vi "image process.vi"(0 "Picture in":refnum<vi>, 1 "reference in":refnum<vi>, 4 "XYGraph Refnum":refnum<vi>, 5 "error in (no error)":errorcluster, 6 "Konverziós faktor":i32 min=0 max=16777215, 7 "picture in":path, 8 "Szürkeárnyalat":i32) -> (10 "new picture 3":picture, 11 "scale maximum":u32, 12 "régi y felbontás":i16, 13 "átméretezett kép":i32[][](array[numeric]), 14 "régi x felbontás":i16, 15 "új y felbontás / sorok száma":i32, 16 "új x felbontás / oszlopok száma":i32, 17 "new picture 2":picture, 19 "error out":errorcluster)   [LabVIEW 2016]
uses:
  <vilib>/Utility/miscctls.llb/LVBoundsTypeDef.ctl
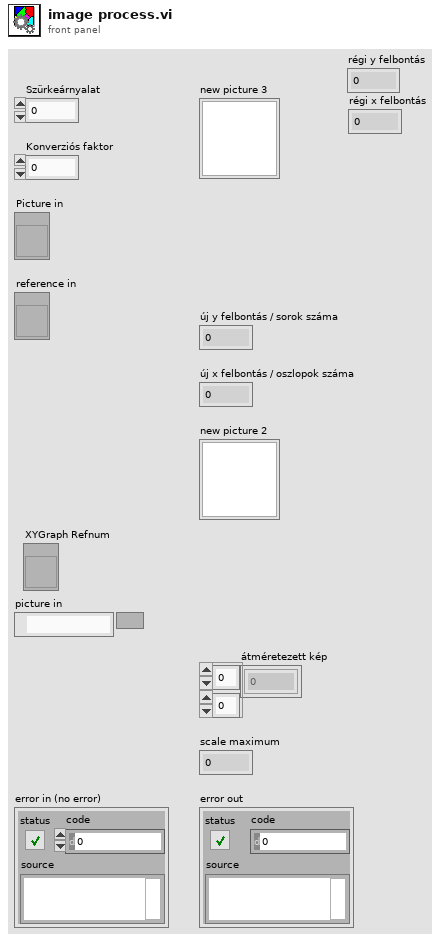
[diagram p1: front panel]
types:
  T1 = typedef "LVBoundsTypeDef.ctl" = cluster{"Width":u32, "Height":u32}
  T2 = typedef "imagedata.ctl" = cluster{"image type":i32, "image depth":i32, "image":u8[], "mask":u8[], "colors":u32[], "Rectangle":cluster{"left":i16, "top":i16, "right":i16, "bottom":i16}}
  T3 = cluster{"left":i16, "top":i16, "right":i16, "bottom":i16}
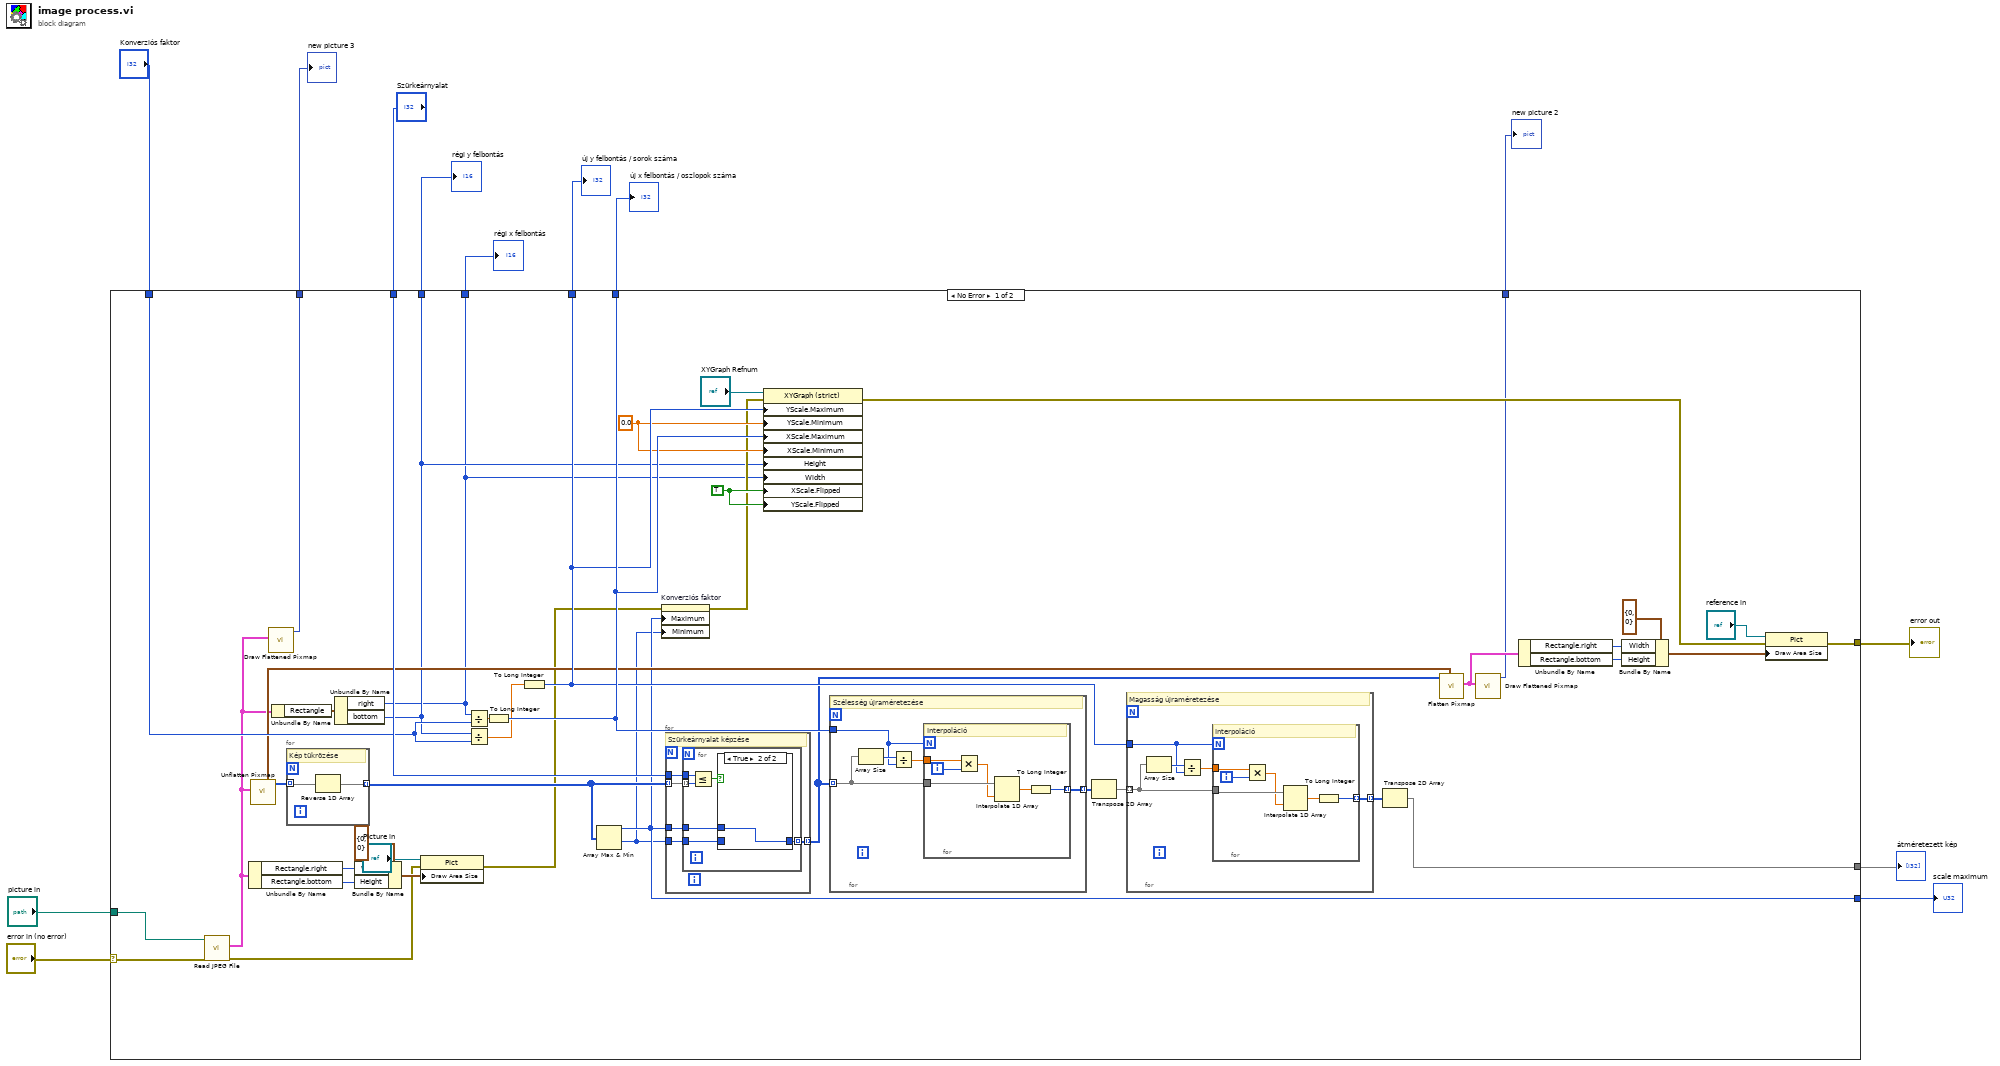
[diagram p0: block diagram]
diagram:
  n1 = case shown="No Error" "error in (no error)" {
    selector: "error in (no error)" -> [w22 w94]
    tunnel: [w16 w94] -> w13
    tunnel: "picture in" -> [w55 _]
    tunnel: [w54 _] -> w11
    tunnel: [w53 _] -> w10
    tunnel: [w52 _] -> w9
    tunnel: [w20 _] -> w8
    tunnel: "Szürkeárnyalat" -> [w50 _]
    tunnel: "Konverziós faktor" -> [w49 _]
    tunnel: [w38 _] -> w5
    tunnel: [w26 _] -> w4
    tunnel: [w15 _] -> w2
    tunnel: [w14 _] -> w1
    frame No Error {
      w51 = TRUE
      w46 = 0.0 ("Y Scale.Range:Minimum")
      n2 = call <vilib>:"Read JPEG File.vi"("error in (no error)"=w22, "path to JPEG file"=w55) -> ("error out"=w21:errorcluster, "image data"=w35:T2)  [unwired: 7 in, 1 out]
      n3 = Unbundle By Name(w35) -> ("Rectangle.right"=w36:i16, "Rectangle.bottom"=w37:i16)
      n4 = call <vilib>:"Unflatten Pixmap.vi"("image data"=w35) -> ("24-bit pixmap"=w47:u32[][], "top left"=w45:cluster{"x":i16, "y":i16})  [unwired: 4 in, 5 out]
      n5 = call <vilib>:"Draw Flattened Pixmap.vi"("image data"=w35) -> ("new picture"=w26:picture)  [unwired: 8 in]
      n6 = Unbundle By Name(w35) -> ("Rectangle"=w30:T3)
      n7 = for {
        tunnel: w47 -> [w58] mode=indexing
        tunnel: [w57] -> w48 mode=indexing
        # "Kép tükrözése"
        n8 = Reverse 1D Array(array=w58) -> (reversed array=w57:u32[])
      }
      n9 = Unbundle By Name(w30) -> ("right"=w14:i16, "bottom"=w15:i16)
      n10 = Bundle By Name(cluster=T1 {"Width"=0, "Height"=0} ("Draw Area Size"), "Width"=w36, "Height"=w37) -> (w34:T1)
      n11 = property on="Property Node" class="Pict"(reference="Picture in", error in=w21, "Draw Area Size"=w34) -> (error out=w17:errorcluster)  [unwired: 1 out]
      n12 = Divide(x=w14, y=w49) -> (x/y=w31:dbl)
      n13 = Divide(x=w15, y=w49) -> (x/y=w32:dbl)
      n14 = To Long Integer(number=w31) -> (32bit integer=w54:i32)
      n15 = To Long Integer(number=w32) -> (32bit integer=w53:i32)
      n16 = Array Max & Min(array=w48) -> (max value=w20:u32, min value=w19:u32)  [unwired: 2 out]
      n17 = property on="Konverziós faktor" class="DigNum (strict)"(error in=w17, "Maximum"=w20, "Minimum"=w19) -> (error out=w18:errorcluster)  [unwired: 1 in, 1 out]
      n18 = for {
        tunnel: w48 -> [w63] mode=indexing
        tunnel: w50 -> [w62]
        tunnel: w20 -> [w61]
        tunnel: [w60] -> w44 mode=indexing
        tunnel: w19 -> [w59]
        # "Szürkeárnyalat képzése"
        n19 = for {
          tunnel: w63 -> [w68] mode=indexing
          tunnel: w62 -> [w67]
          tunnel: w61 -> [w66]
          tunnel: [w65] -> w60 mode=indexing
          tunnel: w59 -> [w64]
          n20 = Less Or Equal?(x=w67, y=w68) -> (x <= y?=w69:bool)
          n21 = case shown="True" w69 {
            tunnel: w66 -> [_ w71]
            tunnel: [w70 w71] -> w65
            tunnel: w64 -> [w70 _]
            frame False {
            }
            frame True {
            }
          }
        }
      }
      n22 = property on="Property Node" class="XYGraph (strict)"(reference="XYGraph Refnum", error in=w18, "YScale.Maximum"=w53, "YScale.Minimum"=w46, "XScale.Maximum"=w54, "XScale.Minimum"=w46, "Height"=w15, "Width"=w14, "XScale.Flipped"=w51, "YScale.Flipped"=w51) -> (error out=w56:errorcluster)  [unwired: 1 out]
      n23 = for {
        tunnel: w44 -> [w83] mode=indexing
        tunnel: [w85] -> w27 mode=indexing
        tunnel: w54 -> [w84]
        # "Szélesség újraméretezése"
        n24 = Array Size(array=w83) -> (size(s)=w87:i32)
        n25 = Divide(x=w87, y=w84) -> (x/y=w86:dbl)
        n26 = for {
          N: w84 -> [_]
          tunnel: w83 -> [w93]
          tunnel: w86 -> [w91]
          tunnel: [w88] -> w85 mode=indexing
          i -> [w92]
          # "Interpoláció"
          n27 = Multiply(x=w91, y=w92) -> (x*y=w90:dbl)
          n28 = Interpolate 1D Array(1:w90, 2:w93) -> (0:w89:dbl)
          n29 = To Long Integer(number=w89) -> (32bit integer=w88:i32)
        }
      }
      n30 = Transpose 2D Array(2D array=w27) -> (transposed array=w28:i32[][])
      n31 = for {
        tunnel: w28 -> [w72] mode=indexing
        tunnel: [w74] -> w29 mode=indexing
        tunnel: w53 -> [w73]
        # "Magasság újraméretezése"
        n32 = Array Size(array=w72) -> (size(s)=w76:i32)
        n33 = Divide(x=w76, y=w73) -> (x/y=w75:dbl)
        n34 = for {
          N: w73 -> [_]
          tunnel: w72 -> [w82]
          tunnel: w75 -> [w80]
          tunnel: [w77] -> w74 mode=indexing
          i -> [w81]
          # "Interpoláció"
          n35 = Multiply(x=w80, y=w81) -> (x*y=w79:dbl)
          n36 = Interpolate 1D Array(1:w79, 2:w82) -> (0:w78:dbl)
          n37 = To Long Integer(number=w78) -> (32bit integer=w77:i32)
        }
      }
      n38 = Transpose 2D Array(2D array=w29) -> (transposed array=w52:i32[][])
      n39 = call <vilib>:"Flatten Pixmap.vi"("top left"=w45, "24-bit pixmap"=w44) -> ("image data"=w43:T2)  [unwired: 9 in]
      n40 = call <vilib>:"Draw Flattened Pixmap.vi"("image data"=w43) -> ("new picture"=w38:picture)  [unwired: 8 in]
      n41 = Unbundle By Name(w43) -> ("Rectangle.right"=w40:i16, "Rectangle.bottom"=w39:i16)
      n42 = Bundle By Name(cluster=T1 {"Width"=0, "Height"=0} ("Draw Area Size"), "Width"=w40, "Height"=w39) -> (w42:T1)
      n43 = property on="Property Node" class="Pict"(reference="reference in", error in=w56, "Draw Area Size"=w42) -> (error out=w16:errorcluster)  [unwired: 1 out]
    }
    frame Error {
    }
  }
  "error out" <- w13
  "új x felbontás / oszlopok száma" <- w11
  "új y felbontás / sorok száma" <- w10
  "átméretezett kép" <- w9
  "scale maximum" <- w8
  "new picture 2" <- w5
  "new picture 3" <- w4
  "régi y felbontás" <- w2
  "régi x felbontás" <- w1
